vi "CrossedLine.vi"(0 "Xpoint1":dbl, 1 "Ypoint1":dbl, 4 "Xpoint2":dbl, 5 "Ypoint2":dbl, 6 "XpointC":dbl, 7 "YpointC":dbl, 8 "XpointP":dbl=-1.0, 9 "YpointP":dbl=-1.0) -> (12 "NextPriorX":dbl, 13 "NextPriorY":dbl, 17 "CrossedLine":bool)   [LabVIEW 2012]
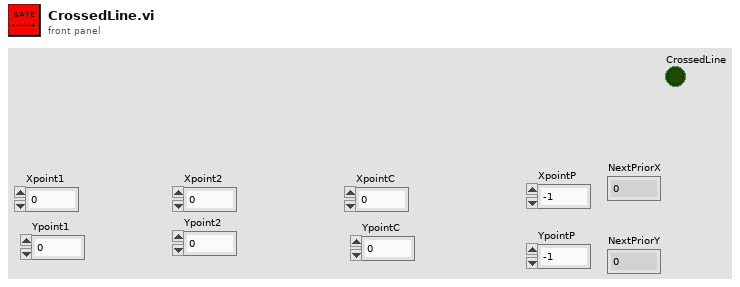
[diagram p1: front panel]
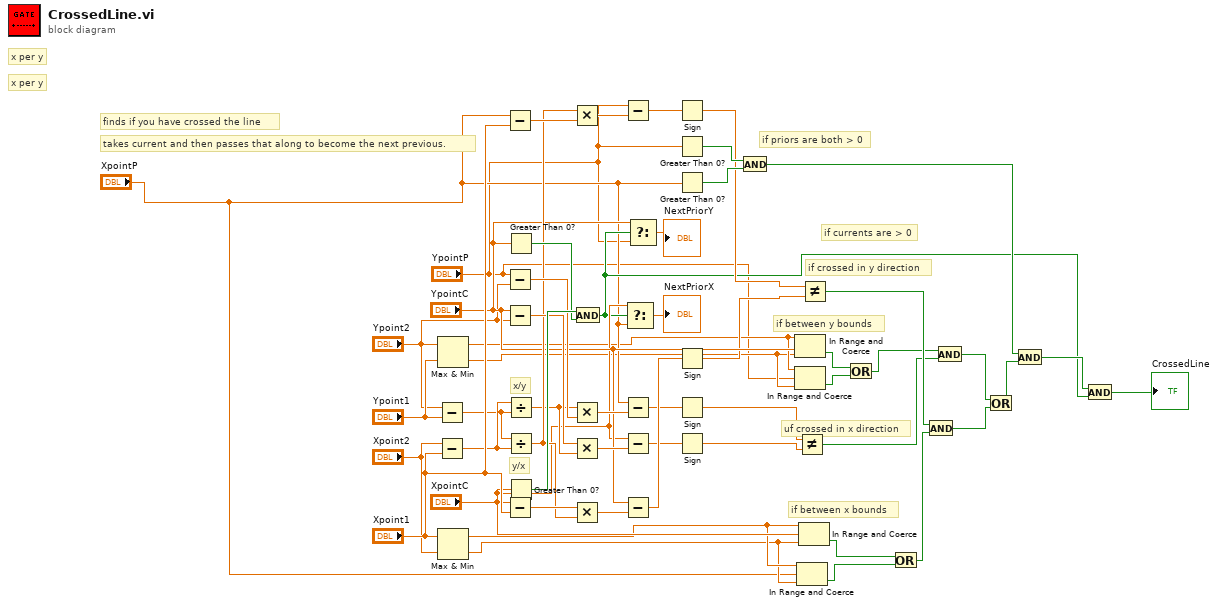
[diagram p0: block diagram]
diagram:
  # "if currents are > 0"
  # "uf crossed in x direction"
  # "if crossed in y direction"
  # "y/x"
  # "x/y"
  # "if between x bounds"
  # "if between y bounds"
  # "if priors are both > 0"
  # "x per y"
  # "finds if you have crossed the line"
  # "takes current and then passes that along to become the next previous."
  # "x per y"
  n1 = Subtract(x="Ypoint2", y="Ypoint1") -> (x-y=w28:dbl)
  n2 = Subtract(x="Xpoint2", y="Xpoint1") -> (x-y=w29:dbl)
  n3 = Max & Min(x="Ypoint2", y="Ypoint1") -> (max(x,y)=w6:dbl, min(x,y)=w5:dbl)
  n4 = Max & Min(x="Xpoint1", y="Xpoint2") -> (max(x,y)=w12:dbl, min(x,y)=w11:dbl)
  n5 = Subtract(x="XpointP", y="Xpoint1") -> (x-y=w52:dbl)
  n6 = Subtract(x="YpointP", y="Ypoint2") -> (x-y=w39:dbl)
  n7 = Subtract(x="YpointC", y="Ypoint2") -> (x-y=w40:dbl)
  n8 = Subtract(x="XpointC", y="Xpoint1") -> (x-y=w53:dbl)
  n9 = Greater Than 0?(x="YpointC") -> (x > 0?=w42:bool)
  n10 = Divide(x=w29, y=w28) -> (x/y=w27:dbl)
  n11 = Divide(x=w28, y=w29) -> (x/y=w32:dbl)
  n12 = Greater Than 0?(x="XpointC") -> (x > 0?=w43:bool)
  n13 = Multiply(x=w32, y=w52) -> (x*y=w50:dbl)
  n14 = Multiply(x=w27, y=w39) -> (x*y=w37:dbl)
  n15 = Multiply(x=w40, y=w27) -> (x*y=w38:dbl)
  n16 = Multiply(x=w53, y=w32) -> (x*y=w51:dbl)
  n17 = And(x=w43, y=w42) -> (x .and. y?=w14:bool)
  n18 = Subtract(x="YpointP", y=w50) -> (x-y=w48:dbl)
  n19 = Subtract(x="XpointP", y=w37) -> (x-y=w35:dbl)
  n20 = Subtract(x="XpointC", y=w38) -> (x-y=w36:dbl)
  n21 = Subtract(x="YpointC", y=w51) -> (x-y=w49:dbl)
  n22 = Select(t="XpointC", s=w14, f="XpointP") -> (s? t:f=→"NextPriorX":dbl)
  n23 = Select(t="YpointC", s=w14, f="YpointP") -> (s? t:f=→"NextPriorY":dbl)
  n24 = Sign(1:w48) -> (0:w25:dbl)
  n25 = Greater Than 0?(x="YpointP") -> (x > 0?=w44:bool)
  n26 = Greater Than 0?(x="XpointP") -> (x > 0?=w45:bool)
  n27 = Sign(1:w49) -> (0:w24:dbl)
  n28 = Sign(1:w35) -> (0:w22:dbl)
  n29 = Sign(1:w36) -> (0:w23:dbl)
  n30 = And(x=w44, y=w45) -> (x .and. y?=w16:bool)
  n31 = In Range and Coerce(upper limit=w6, x="YpointC", lower limit=w5) -> (In Range?=w3:bool)  [unwired: 1 out]
  n32 = In Range and Coerce(upper limit=w6, x="YpointP", lower limit=w5) -> (In Range?=w2:bool)  [unwired: 1 out]
  n33 = Not Equal?(x=w22, y=w23) -> (x != y?=w20:bool)
  n34 = In Range and Coerce(upper limit=w12, x="XpointP", lower limit=w11) -> (In Range?=w9:bool)  [unwired: 1 out]
  n35 = In Range and Coerce(upper limit=w12, x="XpointC", lower limit=w11) -> (In Range?=w8:bool)  [unwired: 1 out]
  n36 = Not Equal?(x=w25, y=w24) -> (x != y?=w21:bool)
  n37 = Or(x=w3, y=w2) -> (x .or. y?=w1:bool)
  n38 = Or(x=w8, y=w9) -> (x .or. y?=w7:bool)
  n39 = And(x=w21, y=w7) -> (x .and. y?=w19:bool)
  n40 = And(x=w1, y=w20) -> (x .and. y?=w18:bool)
  n41 = Or(x=w18, y=w19) -> (x .or. y?=w17:bool)
  n42 = And(x=w16, y=w17) -> (x .and. y?=w15:bool)
  n43 = And(x=w15, y=w14) -> (x .and. y?=→"CrossedLine":bool)
